vi "VerifyArguments.vi"(8 "error in (no error)":errorcluster, 11 "UniquifyFullyQualifiedVIName in":refnum<class "UniquifyFullyQualifiedVIName.lvclass">) -> (0 "error out":errorcluster, 3 "UniquifyFullyQualifiedVIName out":refnum<class "UniquifyFullyQualifiedVIName.lvclass">)   [LabVIEW 2015, in "UniquifyFullyQualifiedVIName.lvclass"]
uses:
  UniquifyFullyQualifiedVIName.lvclass
  UniquifyFullyQualifiedVIName.lvclass/UniquifyFullyQualifiedVIName.ctl
  <nishared>/LabVIEW CLI/Operations/Utilities/OperationErrorType.ctl
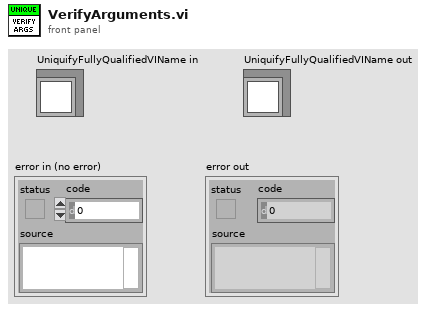
[diagram p1: front panel]
types:
  T1 = typedef "OperationErrorType.ctl" = enum16{"RequiredArgumentMissing", "UnknownArguments", "LoggerSetMultipleTimes", "OperationBrokenError"}
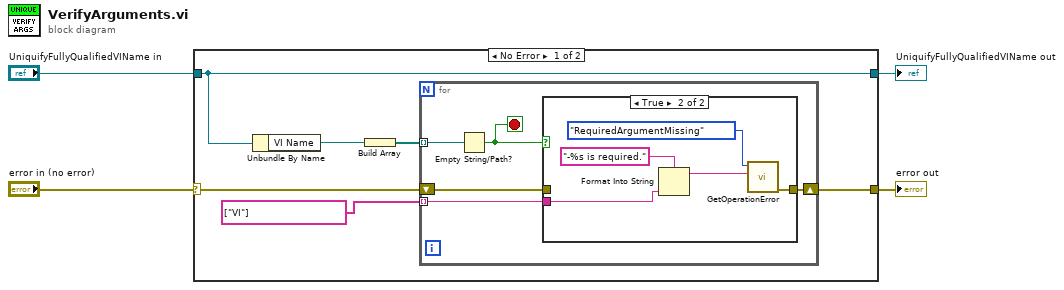
[diagram p0: block diagram]
diagram:
  n1 = case shown="No Error" "error in (no error)" {
    selector: "error in (no error)" -> [w10 w23]
    tunnel: [w9 w23] -> w4
    tunnel: [w8 w22] -> w1
    tunnel: "UniquifyFullyQualifiedVIName in" -> [w8 w22]
    frame No Error {
      n2 = Unbundle By Name(w8) -> ("VI Name"=w6:path)
      n3 = Build Array(w6) -> (w5:path[])
      n4 = for {
        shift-right: [w14] -> w9
        shift-left: w10 -> [w15]
        tunnel: string[] ["VI"] ("Additional Information") -> [w13] mode=indexing
        tunnel: w5 -> [w12] mode=indexing
        stop <- w11 stop-if-true
        n5 = Empty String/Path?(string/path=w12) -> (empty?=w11:bool)
        n6 = case shown="True" w11 {
          tunnel: w15 -> [w16 _]
          tunnel: [w16 w21] -> w14
          tunnel: w13 -> [_ w17]
          frame False {
          }
          frame True {
            n7 = Format Into String(format string="-%s is required.", w17) -> (resulting string=w18:string)  [unwired: 2 in, 1 out]
            n8 = call <nishared>:"GetOperationError.vi"("Additional Information"=w18, "Operation Error Type"=OperationErrorType."RequiredArgumentMissing") -> ("error out"=w21:errorcluster)  [unwired: 9 in]
          }
        }
      }
    }
    frame Error {
    }
  }
  "error out" <- w4
  "UniquifyFullyQualifiedVIName out" <- w1
